vi "SVGlobal_WriteStat.vi"() -> ()   [LabVIEW 2020, in "Shared Variable Interface.lvlib"]
uses:
  Shared Variable Interface.lvlib
panel:
  in  "WriteRate":dbl
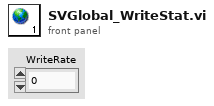
[diagram p1: front panel]
diagram:
